vi "zero.out.and.convert.vi"(11 "data":T1={"enabled"=[TRUE, TRUE, TRUE, TRUE, TRUE, TRUE, TRUE, TRUE], "byte"=[0, 0, 0, 0, 0, 0, 0, 0]} {"byte" format="%.0x"}) -> (2 "u64.be":u64 format="%.0x", 3 "Num.of.True":u8)   [LabVIEW 2020]
uses:
  bats.parser/data.ctl
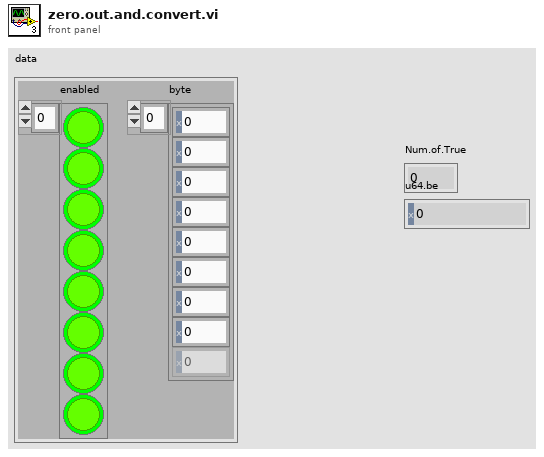
[diagram p1: front panel]
types:
  T1 = typedef "data.ctl" = cluster{"enabled":bool[], "byte":u8[]}
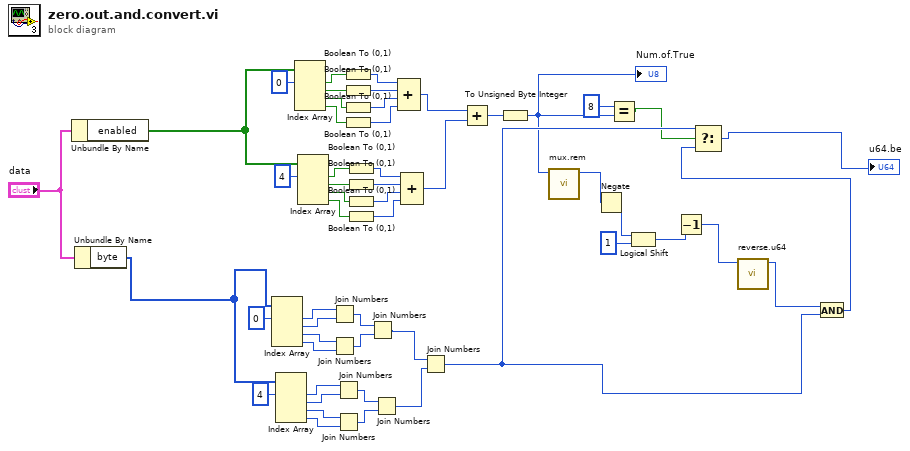
[diagram p0: block diagram]
diagram:
  n1 = Unbundle By Name("data") -> ("enabled"=w31:bool[])
  n2 = Unbundle By Name("data") -> ("byte"=w13:u8[])
  n3 = Index Array(array=w13, index #1=0 ("index")) -> (element #1=w28:u8, element #2=w27:u8, element #3=w26:u8, element #4=w25:u8)  [unwired: 3 in]
  n4 = Index Array(array=w13, index #1=4 ("index")) -> (element #1=w20:u8, element #2=w19:u8, element #3=w18:u8, element #4=w17:u8)  [unwired: 3 in]
  n5 = Index Array(array=w31, index #1=0 ("index")) -> (element #1=w33:bool, element #2=w35:bool, element #3=w37:bool, element #4=w40:bool)  [unwired: 3 in]
  n6 = Index Array(array=w31, index #1=4 ("index")) -> (element #1=w43:bool, element #2=w45:bool, element #3=w47:bool, element #4=w50:bool)  [unwired: 3 in]
  n7 = Join Numbers(hi=w28, lo=w27) -> ((hi.lo)=w24:u16)
  n8 = Join Numbers(hi=w26, lo=w25) -> ((hi.lo)=w23:u16)
  n9 = Join Numbers(hi=w20, lo=w19) -> ((hi.lo)=w16:u16)
  n10 = Join Numbers(hi=w18, lo=w17) -> ((hi.lo)=w15:u16)
  n11 = Boolean To (0,1)(Boolean=w33) -> (0, 1=w34:i16)
  n12 = Boolean To (0,1)(Boolean=w35) -> (0, 1=w36:i16)
  n13 = Boolean To (0,1)(Boolean=w37) -> (0, 1=w38:i16)
  n14 = Boolean To (0,1)(Boolean=w40) -> (0, 1=w39:i16)
  n15 = Boolean To (0,1)(Boolean=w43) -> (0, 1=w44:i16)
  n16 = Boolean To (0,1)(Boolean=w45) -> (0, 1=w46:i16)
  n17 = Boolean To (0,1)(Boolean=w47) -> (0, 1=w48:i16)
  n18 = Boolean To (0,1)(Boolean=w50) -> (0, 1=w49:i16)
  n19 = Join Numbers(hi=w24, lo=w23) -> ((hi.lo)=w22:u32)
  n20 = Join Numbers(hi=w16, lo=w15) -> ((hi.lo)=w14:u32)
  n21 = Compound Arithmetic op=ADD(w34, w36, w38, w39) -> (w41:i16)
  n22 = Compound Arithmetic op=ADD(w44, w46, w48, w49) -> (w51:i16)
  n23 = Join Numbers(hi=w22, lo=w14) -> ((hi.lo)=w4:u64)
  n24 = Add(x=w41, y=w51) -> (x+y=w52:i16)
  n25 = To Unsigned Byte Integer(number=w52) -> (unsigned 8bit integer=w3:u8)
  "Num.of.True" <- w3
  n26 = call "mux.rem.vi"("# of existing\nitems 3"=w3) -> ("y"=w10:i8)  [unwired: 10 in]
  n27 = Negate(x=w10) -> (-x=w9:i8)
  n28 = Equal?(x=u8 8, y=w3) -> (x = y?=w2:bool)
  n29 = Logical Shift(y=w9, x=u64 1) -> (x << y=w12:u64)
  n30 = Decrement(x=w12) -> (x-1=w8:u64)
  n31 = call "reverse.u64.vi"("U64.in"=w8) -> ("U64.reversed"=w7:u64)  [unwired: 10 in]
  n32 = And(x=w7, y=w4) -> (x .and. y?=w5:u64)
  n33 = Select(t=w4, s=w2, f=w5) -> (s? t:f=→"u64.be":u64)
